vi "add error string index_array.vi"(8 "error in (no error)":errorcluster caption="에러 입력(에러 없음)", 10 "index_array":cluster{"start":u32, "end":u32}[](array[cluster]), 11 "Script Line 입력":refnum<class "Script Line.lvclass">) -> (0 "error out":errorcluster caption="에러 출력", 3 "Script Line 출력":refnum<class "Script Line.lvclass">)   [LabVIEW 2020, in "Script Line.lvclass"]
uses:
  Script Line.lvclass
  Script Line.lvclass/Script Line.ctl
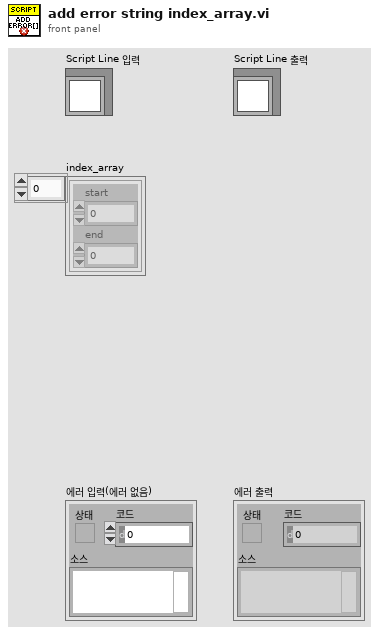
[diagram p1: front panel]
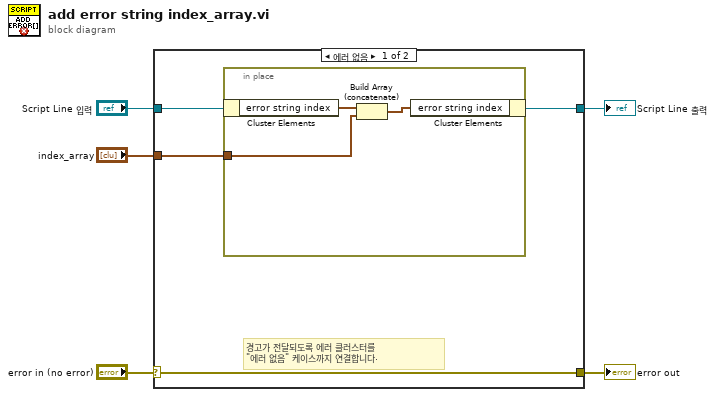
[diagram p0: block diagram]
diagram:
  n1 = case shown="에러 없음" "error in (no error)" {
    selector: "error in (no error)" -> [w9 w14]
    tunnel: [w9 w14] -> w4
    tunnel: [w7 w13] -> w2
    tunnel: "Script Line 입력" -> [w8 w13]
    tunnel: "index_array" -> [w6 _]
    frame No Error {
      # "경고가 전달되도록 에러 클러스터를\n\"에러 없음\" 케이스까지 연결합니다."
      n2 = in-place {
        in-place-border: w6 -> [w10]
        n3 = in-place-cluster #1(w8) -> ("error string index"=w12:cluster{"start":u32, "end":u32}[])
        n4 = Build Array (concatenate)(w12, w10) -> (w11:cluster{"start":u32, "end":u32}[])
        n5 = in-place-cluster #1("error string index"=w11) -> (w7:refnum<class "Script Line.lvclass">)
      }
    }
    frame Error {
    }
  }
  "error out" <- w4
  "Script Line 출력" <- w2
